vi "Control Panel.vi"(8 "error in (no error)":errorcluster, 11 "Spectrometer iHR320 in":refnum<class "Spectrometer iHR320.lvclass">) -> (0 "error out":errorcluster, 3 "Spectrometer iHR320 out":refnum<class "Spectrometer iHR320.lvclass">)   [LabVIEW 2012, in "Spectrometer iHR320.lvclass"]
doc: "(Dynamic) A user-level application that simulates the physical front panel of the Instrument. Provide the user with buttons to manually control features of the instrument, and provide indicators of its current state."
uses:
  Spectrometer iHR320.lvclass
  Spectrometer iHR320.lvclass/Spectrometer iHR320.ctl
  Utility Classes/Scannable/Scannable.lvclass
panel:
  in  "Set Filter":bool
  out "Filter Index":i32(ring)=1 items=["Filter 1"=1, "Empty"=2, "Empty"=3, "Empty"=4, "Filter 2"=5, "Filter 3"=6]
  in  "Filter Index Set":i32(ring)=1 items=["Filter 1"=1, "Empty"=2, "Empty"=3, "Empty"=4, "Filter 2"=5, "Filter 3"=6]
  in  "Copy actual to set":bool
  in  "Populate fields with member data":bool
  out "Grating":u16(ring)=1 items=["1200"=1, "600"=2]
  in  "Set Grating":bool
  in  "stop":bool
  in  "Read to control":bool
  in  "Read":bool
  in  "Go To Wavelength":bool
  in  "Set Slit":bool
  in  "Grating set":u16(ring)=1 items=["1200"=1, "600"=2]
  out "Wavelength":dbl[unit]
  in  "Wavelength Set":dbl[unit]
  out "Exit Slit":dbl[unit]
  in  "Exit Slit Set":dbl[unit]
  out "Entrance Slit":dbl[unit]
  in  "Entrance  set":dbl[unit]
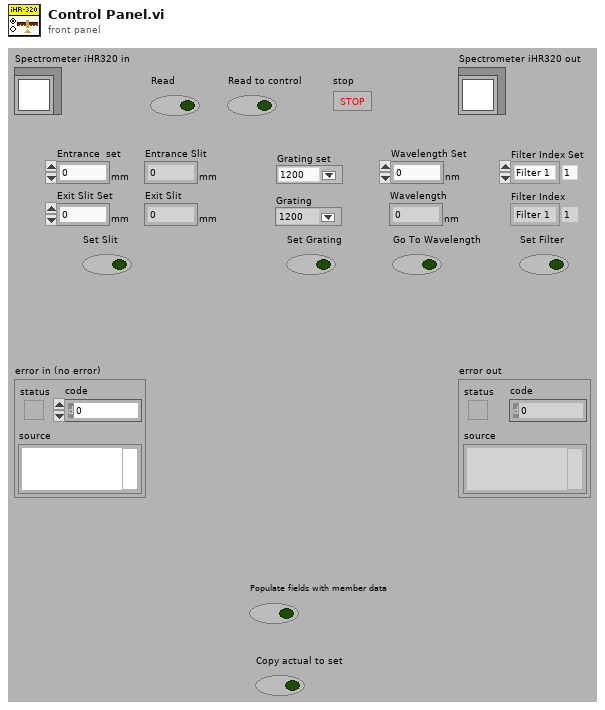
[diagram p1: front panel]
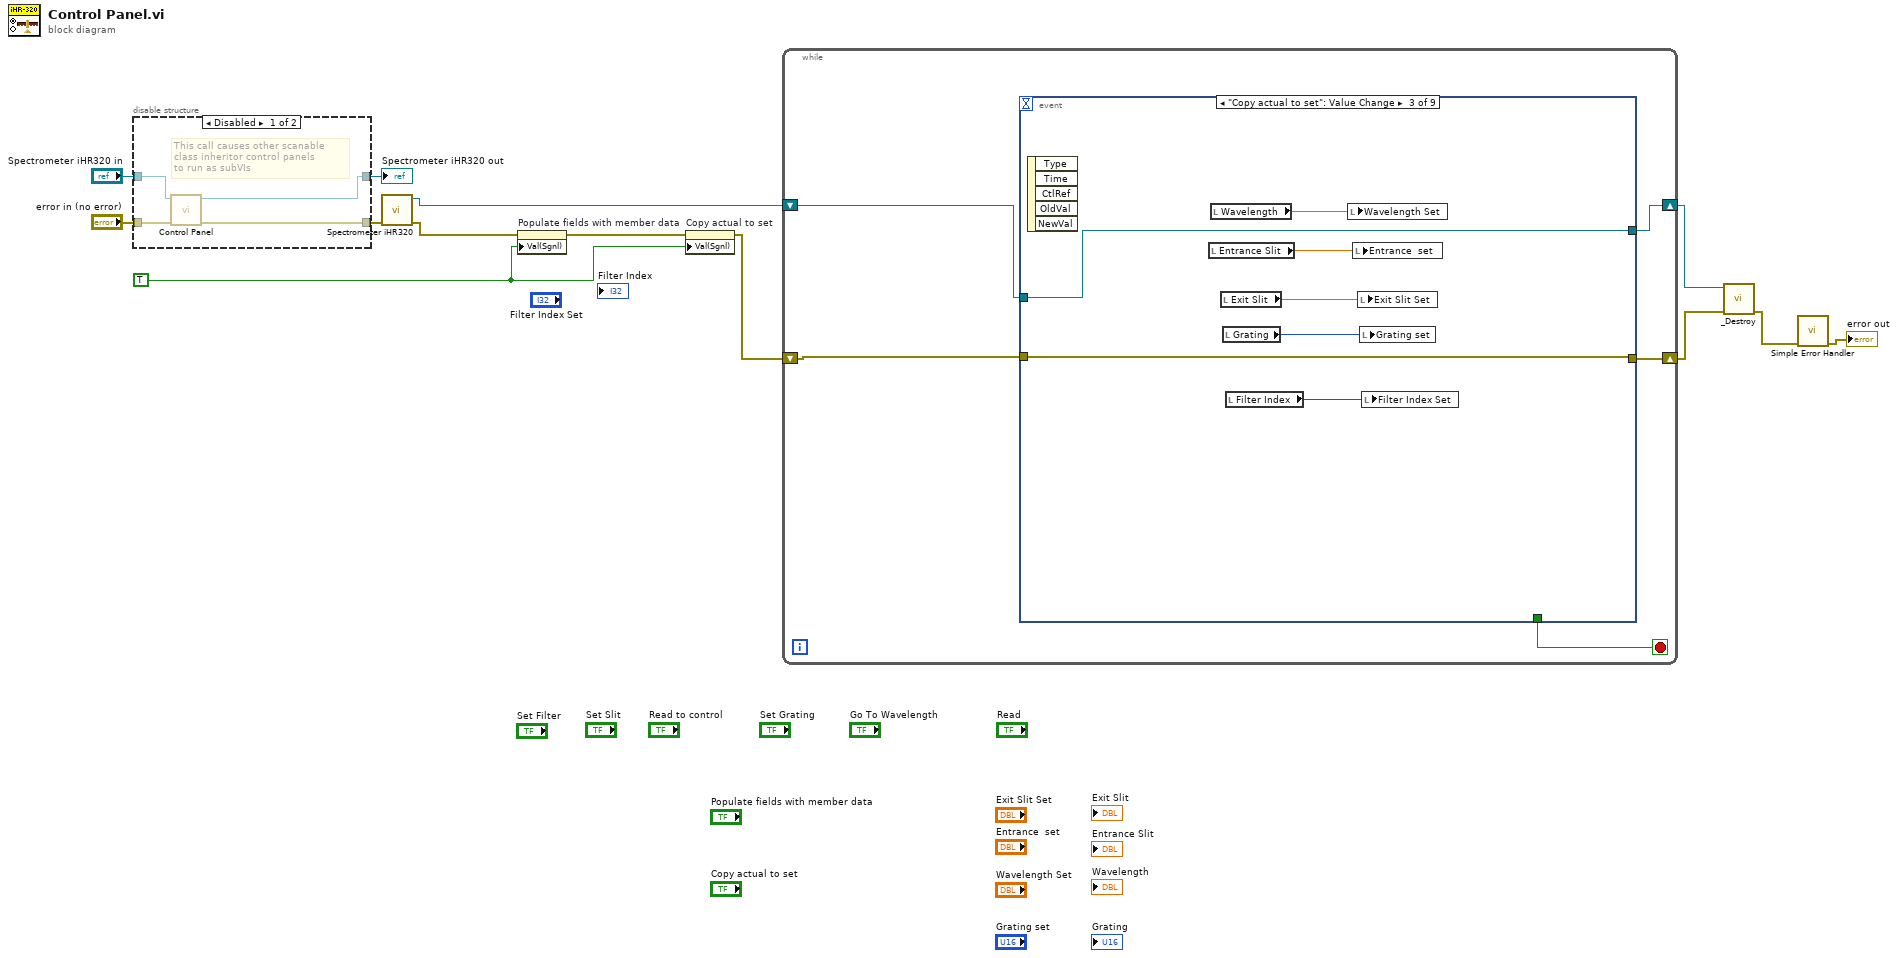
[diagram p0: block diagram]
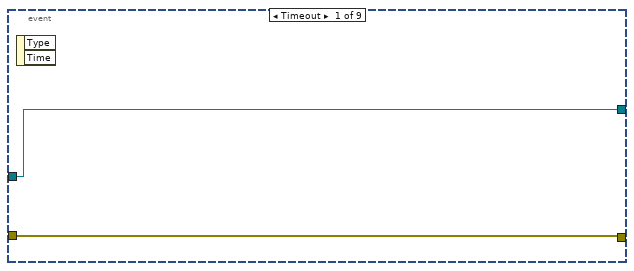
[diagram p3: hidden frame]
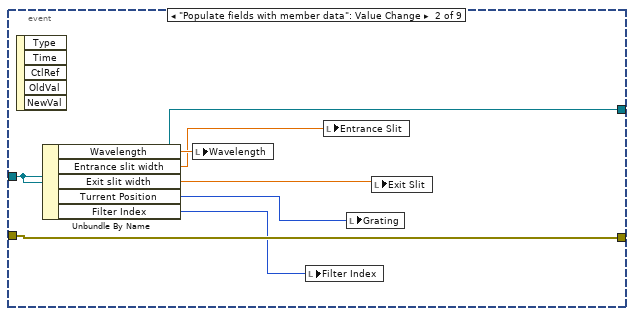
[diagram p4: hidden frame]
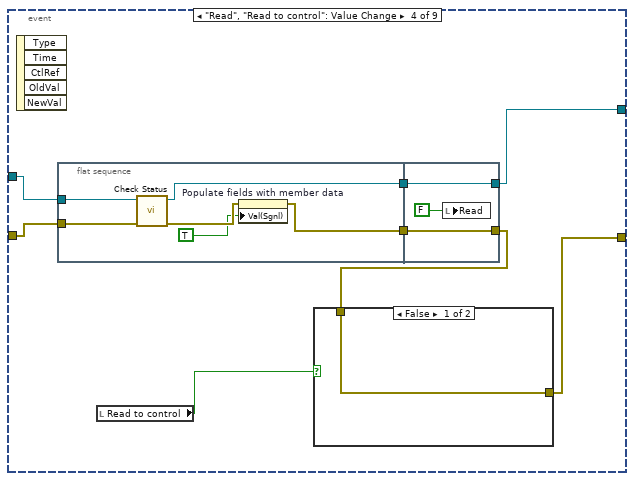
[diagram p5: hidden frame]
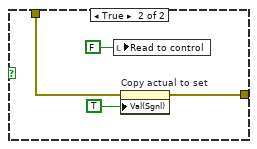
[diagram p6: hidden frame]
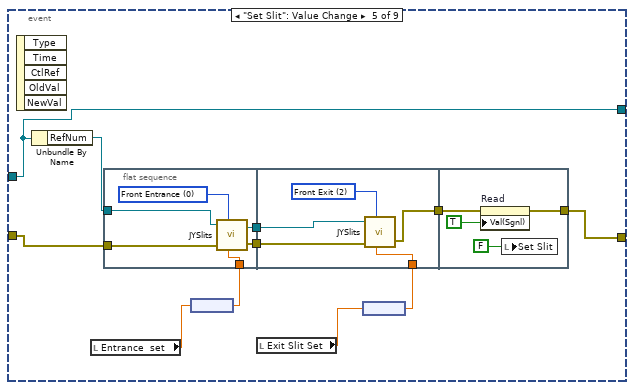
[diagram p7: hidden frame]
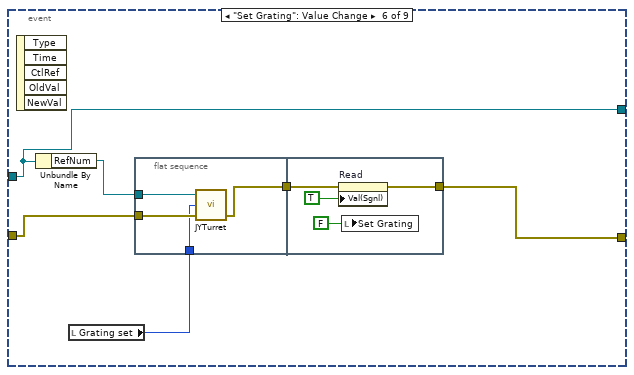
[diagram p8: hidden frame]
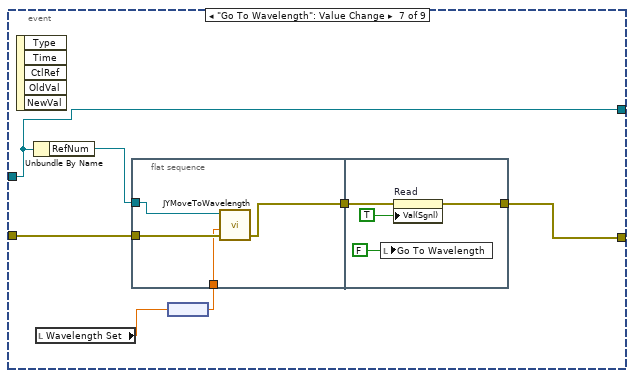
[diagram p9: hidden frame]
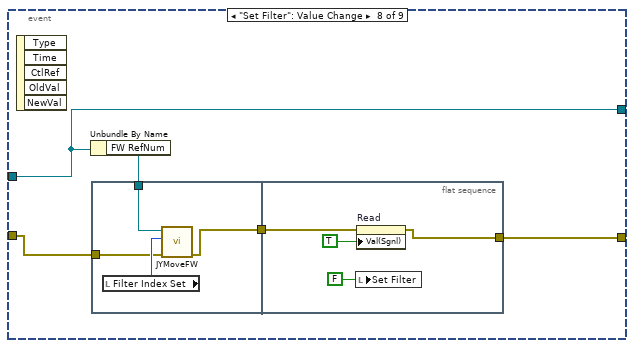
[diagram p10: hidden frame]
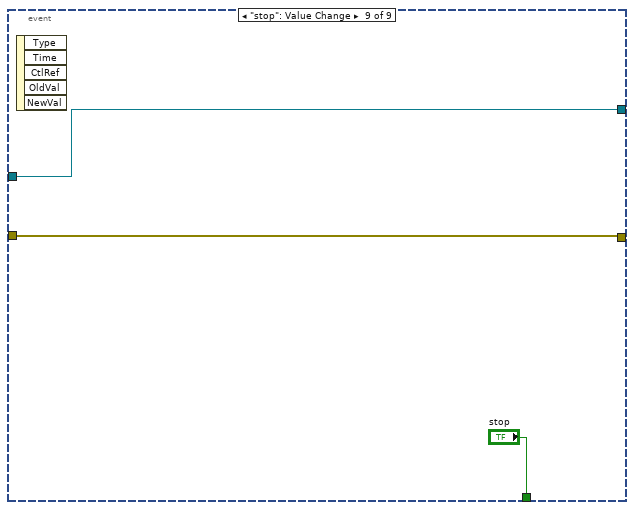
[diagram p11: hidden frame]
diagram:
  w7 = TRUE ("Value (Signaling)")
  n1 = disable-structure shown="Disabled" {
    disable-tunnel: [w17 w19] -> w13
    disable-tunnel: "error in (no error)" -> [w16 w18]
    disable-tunnel: "Spectrometer iHR320 in" -> [w15 w19]
    disable-tunnel: [w14 w18] -> w10
    frame Disabled {
      # "This call causes other scanable\nclass inheritor control panels\nto run as subVIs"
      n2 = call-parent "Control Panel.vi"("error in (no error)"=w16, "Instrument in"=w15) -> ("error out"=w14:errorcluster, "Instrument out"=w17:refnum<class "Spectrometer iHR320.lvclass">)  [unwired: 8 in]
    }
    frame Enabled {
    }
  }
  "Spectrometer iHR320 out" <- w13
  n3 = call "Spectrometer iHR320.vi"("error in (no error)"=w10) -> ("error out"=w9:errorcluster, "Spectr. iHR320 Out"=w5:refnum<class "Spectrometer iHR320.lvclass">)  [unwired: 9 in]
  n4 = property on="Populate fields with member data" class="Bool (strict)"(error in=w9, "Val(Sgnl)"=w7) -> (error out=w8:errorcluster)  [unwired: 1 in, 1 out]
  n5 = property on="Copy actual to set" class="Bool (strict)"(error in=w8, "Val(Sgnl)"=w7) -> (error out=w6:errorcluster)  [unwired: 1 in, 1 out]
  n6 = while {
    shift-right: [w22] -> w2
    shift-left: w6 -> [w24]
    shift-right: [w21] -> w3
    shift-left: w5 -> [w23]
    stop <- w20 stop-if-true
    n7 = event shown="[2] \"Copy actual to set\": Value Change" {
      selector: _ -> [_ _ _ _ _ _ _ _ _]
      dyn-events: _ -> [_ _ _ _ _ _ _ _ _]
      timeout: _ -> [_ _ _ _ _ _ _ _ _]
      tunnel: w24 -> [w26 w29 w35 w48 w70 w93 w109 w120 w133]
      tunnel: w23 -> [w25 w28 w36 w47 w63 w89 w103 w122 w132]
      tunnel: [w26 w29 w35 w42 w71 w91 w104 w118 w133] -> w22
      tunnel: [w25 w28 w36 w41 w63 w89 w103 w122 w132] -> w21
      tunnel: [_ _ _ _ _ _ _ _ "stop"] -> w20
      event Timeout {
        n8 = event-data() -> ()  [unwired: 1 in, 2 out]
      }
      event "Populate fields with member data": Value Change {
        n9 = event-data() -> ()  [unwired: 1 in, 5 out]
        n10 = Unbundle By Name(w28) -> ("Wavelength"=w33:dbl[unit], "Entrance slit width"=w32:dbl[unit], "Exit slit width"=w31:dbl[unit], "Turrent Position"=w30:u16, "Filter Index"=w27:i32)
        n11 = local write "Wavelength"(w33) -> ()
        n12 = local write "Filter Index"(w27) -> ()
        n13 = local write "Entrance Slit"(w32) -> ()
        n14 = local write "Grating"(w30) -> ()
        n15 = local write "Exit Slit"(w31) -> ()
      }
      event "Copy actual to set": Value Change {
        n16 = event-data() -> ()  [unwired: 1 in, 5 out]
        n17 = local read "Entrance Slit"() -> (w39:dbl[unit])
        n18 = local read "Wavelength"() -> (w40:dbl[unit])
        n19 = local read "Exit Slit"() -> (w38:dbl[unit])
        n20 = local read "Grating"() -> (w37:u16)
        n21 = local read "Filter Index"() -> (w34:i32)
        n22 = local write "Wavelength Set"(w40) -> ()
        n23 = local write "Entrance  set"(w39) -> ()
        n24 = local write "Exit Slit Set"(w38) -> ()
        n25 = local write "Grating set"(w37) -> ()
        n26 = local write "Filter Index Set"(w34) -> ()
      }
      event "Read", "Read to control": Value Change {
        n27 = event-data() -> ()  [unwired: 1 in, 5 out]
        n28 = flat-sequence {
          tunnel: w48 -> [w59]
          tunnel: w47 -> [w58]
          tunnel: [w55] -> w46
          tunnel: [w54] -> w45
          tunnel: [w61] -> w43
          tunnel: w46 -> [w61]
          tunnel: [w60] -> w41
          tunnel: w45 -> [w60]
          frame #0 {
            n29 = call-dynamic "Check Status.vi"("error in (no error)"=w59, "Spectrometer iHR320 in"=w58) -> ("error out"=w57:errorcluster, "Spectrometer iHR320 out"=w54:refnum<class "Spectrometer iHR320.lvclass">)  [unwired: 6 in, 2 out]
            n30 = property on="Populate fields with member data" class="Bool (strict)"(error in=w57, "Val(Sgnl)"=TRUE ("Value (Signaling)")) -> (error out=w55:errorcluster)  [unwired: 1 in, 1 out]
          }
          frame #1 {
            n31 = local write "Read"(FALSE ("Read")) -> ()
          }
        }
        n32 = local read "Read to control"() -> (w44:bool)
        n33 = case shown="False" w44 {
          tunnel: w43 -> [w49 w51]
          tunnel: [w49 w50] -> w42
          frame False {
          }
          frame True {
            n34 = local write "Read to control"(FALSE ("Read to control")) -> ()
            n35 = property on="Copy actual to set" class="Bool (strict)"(error in=w51, "Val(Sgnl)"=TRUE ("Value (Signaling)")) -> (error out=w50:errorcluster)  [unwired: 1 in, 1 out]
          }
        }
      }
      event "Set Slit": Value Change {
        n36 = event-data() -> ()  [unwired: 1 in, 5 out]
        n37 = Unbundle By Name(w63) -> ("RefNum"=w69:refnum<k7>)
        n38 = local read "Entrance  set"() -> (w67:dbl[unit])
        n39 = flat-sequence {
          tunnel: [w78] -> w73
          tunnel: w70 -> [w77]
          tunnel: w69 -> [w76]
          tunnel: [w75] -> w68
          tunnel: w66 -> [w74]
          tunnel: w73 -> [w83]
          tunnel: [w82] -> w72
          tunnel: w68 -> [w81]
          tunnel: w64 -> [w80]
          tunnel: w72 -> [w86]
          tunnel: [w85] -> w71
          frame #0 {
            w79 = u16 0 items=["Front Entrance", "Side Entrance", "Front Exit", "Side Exit", "First Intermediate", "Second Intermediate"] ("Slit")
            n40 = call "JYSlits.vi"("JYMONOLib.IJYMonoReqd In"=w76, "Slit"=w79, "error in (no error)"=w77, "Slit Width"=w74) -> ("JYMONOLib.IJYMonoReqd Out"=w75:refnum<k7>, "error out"=w78:errorcluster)  [unwired: 1 in]
          }
          frame #1 {
            w84 = u16 2 items=["Front Entrance", "Side Entrance", "Front Exit", "Side Exit", "First Intermediate", "Second Intermediate"] ("Slit")
            n41 = call "JYSlits.vi"("JYMONOLib.IJYMonoReqd In"=w81, "Slit"=w84, "error in (no error)"=w83, "Slit Width"=w80) -> ("error out"=w82:errorcluster)  [unwired: 1 in, 1 out]
          }
          frame #2 {
            n42 = property on="Read" class="Bool (strict)"(error in=w86, "Val(Sgnl)"=TRUE ("Value (Signaling)")) -> (error out=w85:errorcluster)  [unwired: 1 in, 1 out]
            n43 = local write "Set Slit"(FALSE ("Set Slit")) -> ()
          }
        }
        n44 = node(w67) -> (w66:dbl)
        n45 = local read "Exit Slit Set"() -> (w65:dbl[unit])
        n46 = node(w65) -> (w64:dbl)
      }
      event "Set Grating": Value Change {
        n47 = event-data() -> ()  [unwired: 1 in, 5 out]
        n48 = Unbundle By Name(w89) -> ("RefNum"=w94:refnum<k7>)
        n49 = local read "Grating set"() -> (w90:u16)
        n50 = flat-sequence {
          tunnel: w94 -> [w98]
          tunnel: w93 -> [w97]
          tunnel: [w96] -> w92
          tunnel: w90 -> [w95]
          tunnel: w92 -> [w100]
          tunnel: [w99] -> w91
          frame #0 {
            n51 = call "JYTurret.vi"("error in (no error)"=w97, "Grating Index"=w95, "JYMONOLib.IJYMonoReqd In"=w98) -> ("error out"=w96:errorcluster)  [unwired: 2 out]
          }
          frame #1 {
            n52 = property on="Read" class="Bool (strict)"(error in=w100, "Val(Sgnl)"=TRUE ("Value (Signaling)")) -> (error out=w99:errorcluster)  [unwired: 1 in, 1 out]
            n53 = local write "Set Grating"(FALSE ("Set Grating")) -> ()
          }
        }
      }
      event "Go To Wavelength": Value Change {
        n54 = event-data() -> ()  [unwired: 1 in, 5 out]
        n55 = Unbundle By Name(w103) -> ("RefNum"=w107:refnum<k7>)
        n56 = local read "Wavelength Set"() -> (w106:dbl[unit])
        n57 = flat-sequence {
          tunnel: w109 -> [w113]
          tunnel: [w112] -> w108
          tunnel: w107 -> [w111]
          tunnel: w105 -> [w110]
          tunnel: w108 -> [w115]
          tunnel: [w114] -> w104
          frame #0 {
            n58 = call "JYMoveToWavelength.vi"("error in (no error)"=w113, "Target WL"=w110, "RefNum In"=w111) -> ("error out"=w112:errorcluster)  [unwired: 1 in, 2 out]
          }
          frame #1 {
            n59 = local write "Go To Wavelength"(FALSE ("Go To Wavelength")) -> ()
            n60 = property on="Read" class="Bool (strict)"(error in=w115, "Val(Sgnl)"=TRUE ("Value (Signaling)")) -> (error out=w114:errorcluster)  [unwired: 1 in, 1 out]
          }
        }
        n61 = node(w106) -> (w105:dbl)
      }
      event "Set Filter": Value Change {
        n62 = event-data() -> ()  [unwired: 1 in, 5 out]
        n63 = Unbundle By Name(w122) -> ("FW RefNum"=w121:refnum<k7>)
        n64 = flat-sequence {
          tunnel: w121 -> [w126]
          tunnel: w120 -> [w124]
          tunnel: [w123] -> w119
          tunnel: w119 -> [w128]
          tunnel: [w127] -> w118
          frame #0 {
            n65 = local read "Filter Index Set"() -> (w125:i32)
            n66 = call "JYMoveFW.vi"("error in (no error)"=w124, "Filter Index"=w125, "FW RefNum In"=w126) -> ("error out"=w123:errorcluster)  [unwired: 7 in, 1 out]
          }
          frame #1 {
            n67 = local write "Set Filter"(FALSE ("Set Filter")) -> ()
            n68 = property on="Read" class="Bool (strict)"(error in=w128, "Val(Sgnl)"=TRUE ("Value (Signaling)")) -> (error out=w127:errorcluster)  [unwired: 1 in, 1 out]
          }
        }
      }
      event "stop": Value Change {
        n69 = event-data() -> ()  [unwired: 1 in, 5 out]
      }
    }
  }
  n70 = call-dynamic "_Destroy.vi"("error in (no error)"=w2, "Spectrometer iHR320 in"=w3) -> ("error out"=w1:errorcluster)  [unwired: 9 in]
  n71 = call <vilib>:"Simple Error Handler.vi"("error in (no error)"=w1) -> ("error out"=→"error out":errorcluster)  [unwired: 4 in, 4 out]
